vi "Mouse Up.vi"(7 "Map Model in":refnum<class "Map Model.lvclass">, 8 "error in (no error)":errorcluster, 10 "Position":T1, 11 "Eraser in":refnum<class "Eraser.lvclass">) -> (0 "error out":errorcluster, 3 "Eraser out":refnum<class "Eraser.lvclass">, 5 "Map Model out":refnum<class "Map Model.lvclass">)   [LabVIEW 2020, in "Map Model.lvlib" / "Eraser.lvclass"]
uses:
  Eraser.lvclass
  E:/Project/Labview-Projects/Completed projects/Map Editor/Models/Map Model/Tools/Tool/Tool.lvclass
  E:/Project/Labview-Projects/Completed projects/Map Editor/Models/Map Model/Tools/Undoable Tool/Undoable Tool.lvclass
  <vilib>/Utility/miscctls.llb/LVPoint32TypeDef.ctl
  Map Model/Map Model.lvclass
  Tool/Tool.lvclass/Tool.ctl
  Map Model/Map Model.lvclass/Map Model.ctl
  Undoable Tool/Undoable Tool.lvclass/Undoable Tool.ctl
  Undoable Tool/Undoable Tool.lvclass
  Tool/Tool.lvclass
panel:
  # "NOTICE -- YOU MUST LEAVE THIS NOTICE IN PLACE.\n\nCopyright (c) 2017, LIANG LIU Shawn.Liu.cn@gmail.com\nAll rights reserved.\n\nRedistribution and use in source and binary forms, with or without modification, are permitted provided that the following conditions are met:\n-Redistributions of source code must retain the above copyright notice, this list of conditions and the following disclaimer.\n-Redistributions in binary form must reproduce the above copyright notice, this list of conditions and the following disclaimer in the documentation and/or other materials provided with the distribution.\n-Neither the name of the eLp nor the names of its contributors may be used to endorse or promote products derived from this software without specific prior written permission.\n\nTHIS SOFTWARE IS PROVIDED BY THE COPYRIGHT HOLDERS AND CONTRIBUTORS \"AS IS\" AND ANY EXPRESS OR IMPLIED WARRANTIES, INCLUDING, BUT NOT LIMITED TO, THE IMPLIED WARRANTIES OF MERCHANTABILITY AND FITNESS FOR A PARTICULAR PURPOSE ARE DISCLAIMED. IN NO EVENT SHALL THE COPYRIGHT HOLDER OR CONTRIBUTORS BE LIABLE FOR ANY DIRECT, INDIRECT, INCIDENTAL, SPECIAL, EXEMPLARY, OR CONSEQUENTIAL DAMAGES (INCLUDING, BUT NOT LIMITED TO, PROCUREMENT OF SUBSTITUTE GOODS OR SERVICES; LOSS OF USE, DATA, OR PROFITS; OR BUSINESS INTERRUPTION) HOWEVER CAUSED AND ON ANY THEORY OF LIABILITY, WHETHER IN CONTRACT, STRICT LIABILITY, OR TORT (INCLUDING NEGLIGENCE OR OTHERWISE) ARISING IN ANY WAY OUT OF THE USE OF THIS SOFTWARE, EVEN IF ADVISED OF THE POSSIBILITY OF SUCH DAMAGE."
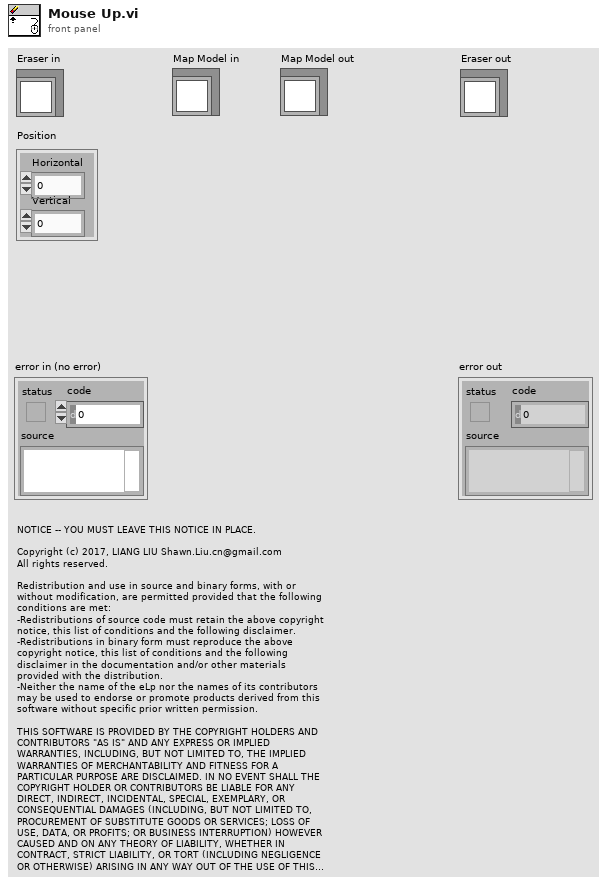
[diagram p1: front panel]
types:
  T1 = typedef "LVPoint32TypeDef.ctl" = cluster{"Horizontal":i32, "Vertical":i32}
  T2 = cluster{"Width":u16, "Style":enum32{"Solid", "Dash", "Dot", "DashDot", "DashDotDot"}}
  T3 = cluster{"Occupied Color":cluster{"Value":u8, "Color":u32}, "Free Color":cluster{"Value":u8, "Color":u32}, "Unknown Color":cluster{"Value":u8, "Color":u32}}
  T4 = typedef "LVPointTypeDef.ctl" = cluster{"Horizontal":i16, "Vertical":i16}
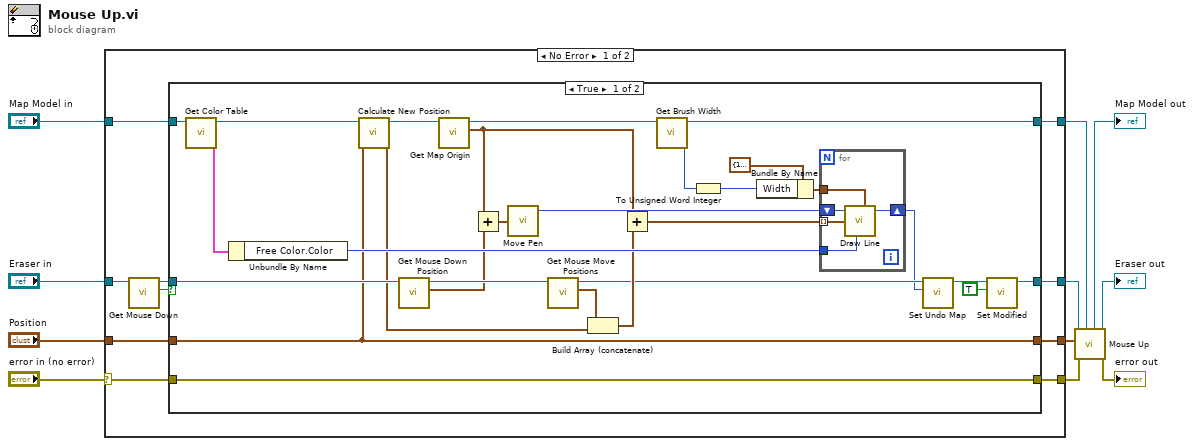
[diagram p0: block diagram]
diagram:
  n1 = case shown="No Error" "error in (no error)" {
    selector: "error in (no error)" -> [w19 w62]
    tunnel: "Map Model in" -> [w21 w61]
    tunnel: "Position" -> [w20 w59]
    tunnel: [w18 w59] -> w7
    tunnel: "Eraser in" -> [w17 w60]
    tunnel: [w16 w60] -> w3
    tunnel: [w15 w62] -> w2
    tunnel: [w14 w61] -> w1
    frame No Error {
      n2 = call "Get Mouse Down.vi"("Tool in"=w17) -> ("Mouse Down"=w12:bool, "Tool out"=w13:refnum<class "Eraser.lvclass">)  [unwired: 9 in]
      n3 = case shown="True" w12 {
        tunnel: w13 -> [w49 w58]
        tunnel: w21 -> [w48 w56]
        tunnel: [w23 w56] -> w14
        tunnel: [w25 w58] -> w16
        tunnel: w20 -> [w26 w55]
        tunnel: [w26 w55] -> w18
        tunnel: w19 -> [w22 w57]
        tunnel: [w22 w57] -> w15
        frame True {
          n4 = call "Get Color Table.vi"("Map Model in"=w48) -> ("Color Table"=w44:T3, "Map Model out"=w45:refnum<class "Map Model.lvclass">)  [unwired: 9 in]
          n5 = Unbundle By Name(w44) -> ("Free Color.Color"=w43:u32)
          n6 = call "Calculate New Position.vi"("Position in"=w26, "Map Model in"=w45) -> ("Position out"=w27:T1, "Map Model out"=w28:refnum<class "Map Model.lvclass">)  [unwired: 8 in]
          n7 = call "Get Mouse Down Position.vi"("Tool in"=w49) -> ("Mouse Down Position"=w38:T1, "Tool out"=w39:refnum<class "Eraser.lvclass">)  [unwired: 9 in]
          n8 = call "Get Map Origin.vi"("Map Model in"=w28) -> ("Map Origin"=w35:T4, "Map Model out"=w40:refnum<class "Map Model.lvclass">)  [unwired: 9 in]
          n9 = Add(x=w35, y=w38) -> (x+y=w37:T1)
          n10 = call <vilib>:"Move Pen.vi"("new position"=w37) -> ("new picture"=w36:picture)  [unwired: 4 in]
          n11 = call "Get Mouse Move Positions.vi"("Tool in"=w39) -> ("Mouse Move Positions"=w29:T1[], "Tool out"=w32:refnum<class "Eraser.lvclass">)  [unwired: 9 in]
          n12 = Build Array (concatenate)(w29, w27) -> (w34:T1[])
          n13 = Add(x=w35, y=w34) -> (x+y=w33:T1[])
          n14 = call "Get Brush Width.vi"("Map Model in"=w40) -> ("Brush Width"=w42:i32, "Map Model out"=w23:refnum<class "Map Model.lvclass">)  [unwired: 9 in]
          n15 = To Unsigned Word Integer(number=w42) -> (unsigned 16bit integer=w41:u16)
          n16 = Bundle By Name(cluster=T2 {"Width"=1, "Style"=enum."Solid"} ("pen"), "Width"=w41) -> (w46:T2)
          n17 = for {
            tunnel: w46 -> [w54]
            tunnel: w43 -> [w53]
            shift-right: [w51] -> w30
            shift-left: w36 -> [w52]
            tunnel: w33 -> [w50] mode=indexing
            n18 = call <vilib>:"Draw Line.vi"("picture"=w52, "end point"=w50, "color(black)"=w53, "pen"=w54) -> ("new picture"=w51:picture)  [unwired: 5 in]
          }
          n19 = call "Set Undo Map.vi"("Undo Map"=w30, "Undoable Tool in"=w32) -> ("Undoable Tool out"=w31:refnum<class "Eraser.lvclass">)  [unwired: 9 in]
          n20 = call "Set Modified.vi"("Modified"=TRUE, "Tool in"=w31) -> ("Tool out"=w25:refnum<class "Eraser.lvclass">)  [unwired: 9 in]
        }
        frame False {
        }
      }
    }
    frame Error {
    }
  }
  n21 = call-parent "Mouse Up.vi"("Map Model in"=w1, "error in (no error)"=w2, "Position"=w7, "Undoable Tool in"=w3) -> ("error out"=→"error out":errorcluster, "Undoable Tool out"=→"Eraser out":refnum<class "Eraser.lvclass">, "Map Model out"=→"Map Model out":refnum<class "Map Model.lvclass">)  [unwired: 5 in]
